vi "Add Request.vi"(8 "error in (no error)":errorcluster, 10 "Write Data":T1, 11 "IP Connection in":refnum<class "IP Connection.lvclass">) -> (0 "error out":errorcluster, 3 "IP Connection out":refnum<class "IP Connection.lvclass">)   [LabVIEW 2011, in "Tinkerforge.lvlib" / "IP Connection.lvclass"]
uses:
  IP Connection.lvclass
  Type Definitions/Message.ctl
  IP Connection.lvclass/IP Connection.ctl
  Type Definitions/Request Identifier.ctl
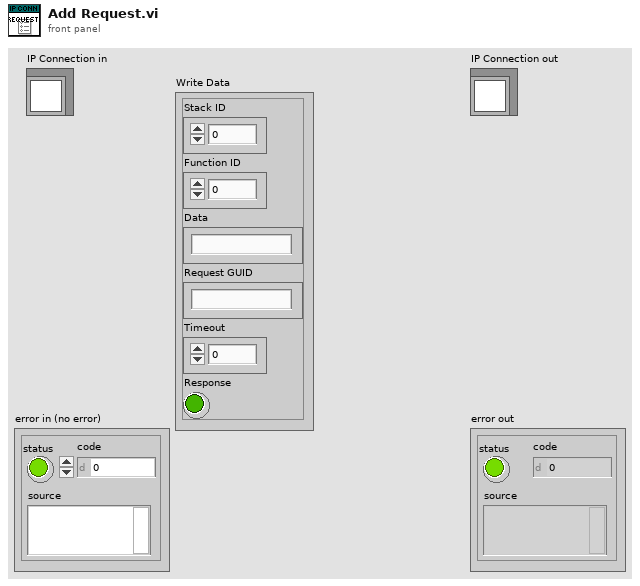
[diagram p1: front panel]
types:
  T1 = typedef "Tinkerforge.lvlib/IP Connection.lvclass/Message.ctl" = cluster{"Stack ID":u8, "Function ID":u8, "Data":string, "Request GUID":string, "Timeout":i32, "Response":bool}
  T2 = typedef "Tinkerforge.lvlib/IP Connection.lvclass/Request Identifier.ctl" = cluster{"Stack ID":u8, "Function ID":u8, "Request GUID":string, "Remaining Timeout":i32}
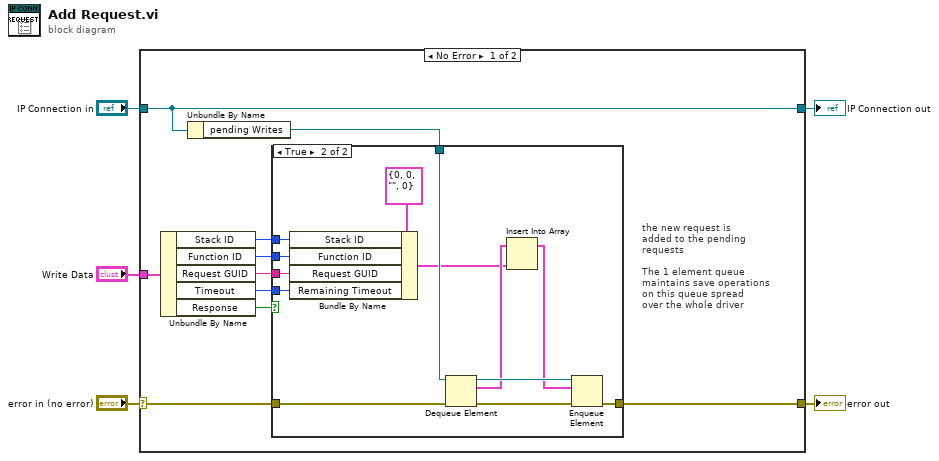
[diagram p0: block diagram]
diagram:
  n1 = case shown="No Error" "error in (no error)" {
    selector: "error in (no error)" -> [w14 w31]
    tunnel: [w7 w31] -> w4
    tunnel: [w15 w30] -> w2
    tunnel: "IP Connection in" -> [w15 w30]
    tunnel: "Write Data" -> [w13 _]
    frame No Error {
      # "the new request is\nadded to the pending\nrequests \n\nThe 1 element queue\nmaintains save operations\non this queue spread\nover the whole driver"
      n2 = Unbundle By Name(w13) -> ("Stack ID"=w12:u8, "Function ID"=w11:u8, "Request GUID"=w10:string, "Timeout"=w9:i32, "Response"=w6:bool)
      n3 = Unbundle By Name(w15) -> ("pending Writes"=w8:refnum<queue>)
      n4 = case shown="True" w6 {
        tunnel: w14 -> [w16 w29]
        tunnel: w12 -> [_ w25]
        tunnel: w11 -> [_ w24]
        tunnel: w10 -> [_ w23]
        tunnel: w9 -> [_ w22]
        tunnel: w8 -> [_ w21]
        tunnel: [w16 w17] -> w7
        frame False {
          # "no response so no answer to wait for"
        }
        frame True {
          n5 = Bundle By Name(cluster=T2 {"Stack ID"=0, "Function ID"=0, "Request GUID"="", "Remaining Timeout"=0} ("new element/subarray"), "Stack ID"=w25, "Function ID"=w24, "Request GUID"=w23, "Remaining Timeout"=w22) -> (w20:T2)
          n6 = Dequeue Element(queue=w21, error in (no error)=w29) -> (queue out=w28:refnum<queue>, element=w27:T2[], error out=w18:errorcluster)  [unwired: 1 in, 1 out]
          n7 = Insert Into Array(array=w27, new element=w20) -> (w19:T2[])  [unwired: 1 in]
          n8 = Enqueue Element(queue=w28, element=w19, error in (no error)=w18) -> (error out=w17:errorcluster)  [unwired: 1 in, 2 out]
        }
      }
    }
    frame Error {
    }
  }
  "error out" <- w4
  "IP Connection out" <- w2
